vi "Actor Core.vi"(8 "error in":errorcluster, 11 "Example GUI Container in":refnum<class "Example GUI Container.lvclass">) -> (0 "error out":errorcluster, 3 "Actor out":refnum<class "Actor.lvclass">)   [LabVIEW 2023, in "Example GUI View.lvlib" / "Example GUI Container.lvclass"]
doc: "(<B>Filename</B>: Actor Framework.lvlib:Actor.lvclass:Actor Core.vi)\n\nReceives messages to the actor, reacts to them, and initiates any error handling that may shut the actor down.\n\nDescendant classes may override this VI to append parallel tasks for the actor to complete while it handles messages. Overrides use the Call Parent Method node."
uses:
  Example GUI Container.lvclass
  <vilib>/ActorFramework/Actor/Actor.lvclass
  <vilib>/ActorFramework/Actor/Actor.lvclass/Actor.ctl
  <vilib>/ActorFramework/Message Enqueuer/Message Enqueuer.lvclass/Message Enqueuer.ctl
  <vilib>/ActorFramework/Message Enqueuer/Init from Existing Queue.vi
  <vilib>/ActorFramework/Message Enqueuer/Enqueue.vi
  <vilib>/ActorFramework/Stop Msg/Stop Msg.lvclass
  <vilib>/Utility/LVClass/Get LV Class Name.vi
  <resource>/AFDebug/Generate Trace for Message.vi
  <vilib>/ActorFramework/Message Priority Queue/Priority Enqueue.vi
  <vilib>/ActorFramework/Message Enqueuer/Message Enqueuer.lvclass
  GUI Views/GUI Container/GUI Container.lvclass
  GUI Views/GUI Container Messages/Insert View into Subpanel Msg/Insert View into Subpanel Msg.lvclass
  GUI Views/GUI Container Messages/Set View FP State Msg/Set View FP State Msg.lvclass
  GUI Views/GUI Container Messages/Open View FP Msg/Open View FP Msg.lvclass
  GUI Views/GUI Container Messages/Close View FP Msg/Close View FP Msg.lvclass
  GUI Views/GUI Container Messages/Remove View from Subpanel Msg/Remove View from Subpanel Msg.lvclass
panel:
  in  "Remove from Subpanel":bool
  in  "Subpanel":string(combo)
  in  "Close Front Panel":bool
  in  "Activate on Open (F)":bool
  in  "Open Front Panel":bool
  in  "Front Panel State":T1(ring)=enum."Standard"
  in  "Set FP State":bool
  in  "Insert in Subpanel":bool
  in  "Exit":bool
  in  "Views":i32(listbox)
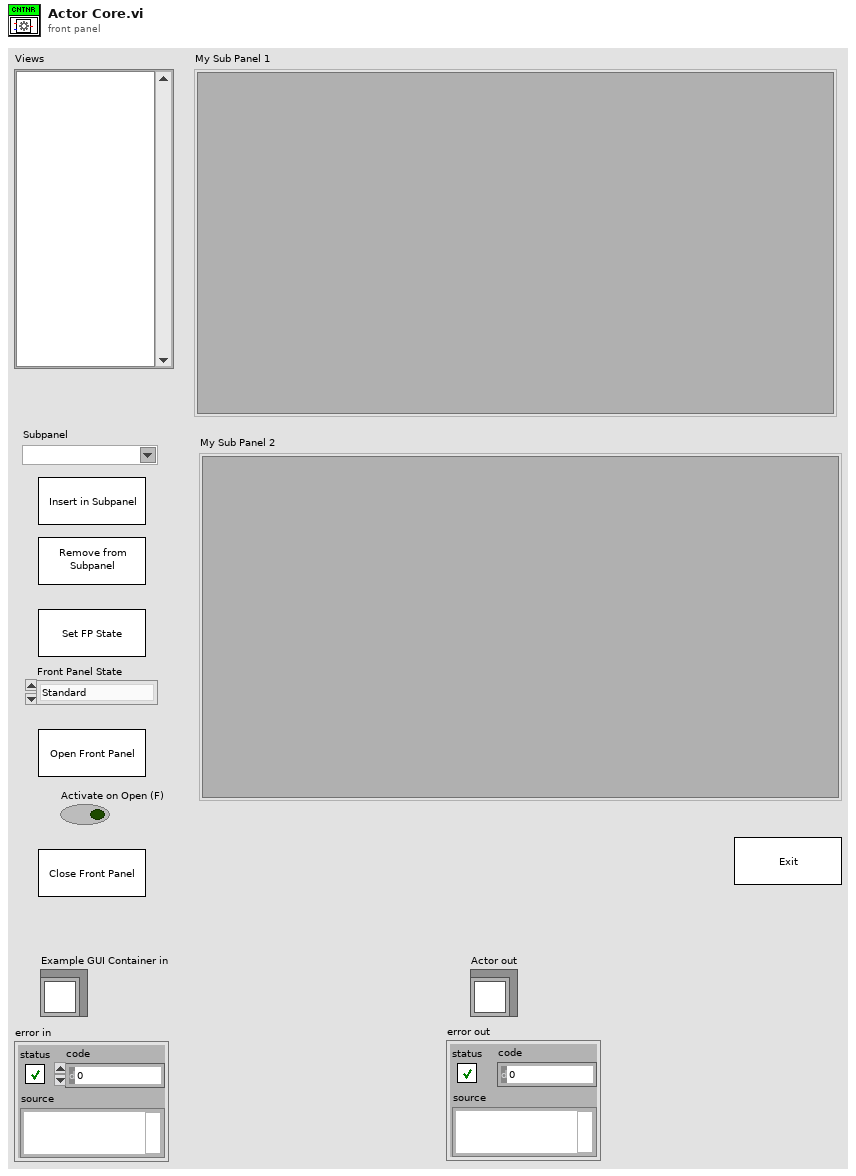
[diagram p1: front panel]
types:
  T1 = enum32{"Invalid", "Standard", "Closed", "Hidden", "Minimized", "Maximized"}
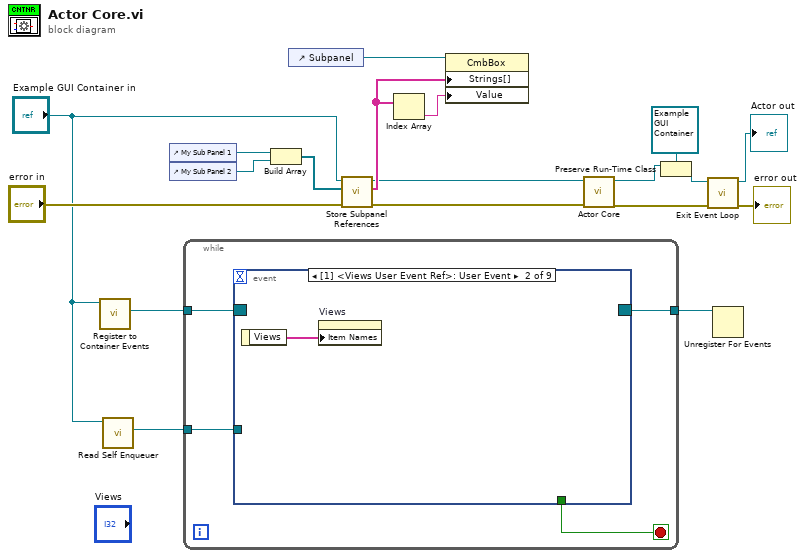
[diagram p0: block diagram]
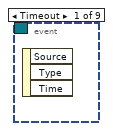
[diagram p2: hidden frame]
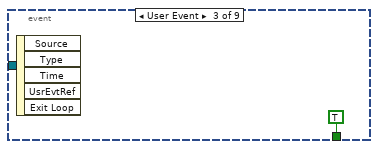
[diagram p3: hidden frame]
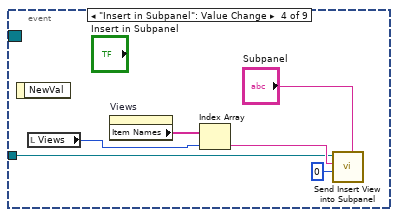
[diagram p4: hidden frame]
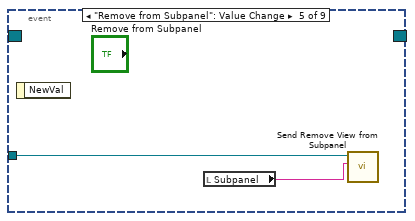
[diagram p5: hidden frame]
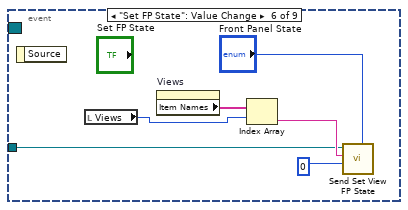
[diagram p6: hidden frame]
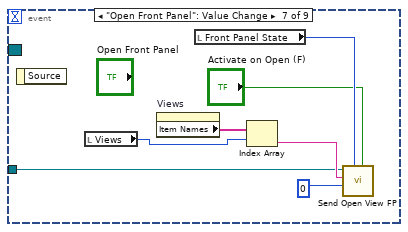
[diagram p7: hidden frame]
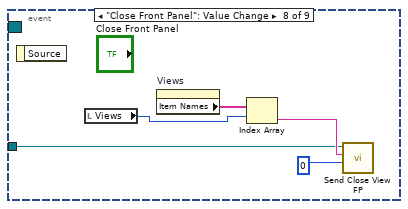
[diagram p8: hidden frame]
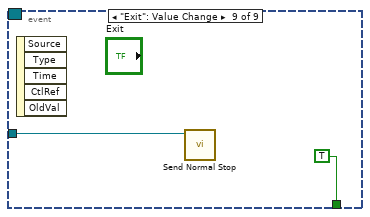
[diagram p9: hidden frame]
diagram:
  n1 = call-dynamic "Register to Container Events.vi"("GUI Container in"="Example GUI Container in") -> ("Event Registration Refnum"=w15:refnum<event-registration>)  [unwired: 8 in, 2 out]
  n2 = call <vilib>:"Read Self Enqueuer.vi"("Actor"="Example GUI Container in") -> ("Self Enqueuer"=w13:refnum<class "Message Enqueuer.lvclass">)  [unwired: 10 in]
  n3 = control-ref of="My Sub Panel 1"() -> (w19:refnum<vi>)
  n4 = control-ref of="My Sub Panel 2"() -> (w11:refnum<vi>)
  n5 = while {
    tunnel: w15 -> [w23]
    tunnel: w13 -> [w22]
    tunnel: [w20] -> w12
    stop <- w21 stop-if-true
    n6 = event shown="[1] <Views User Event Ref>: User Event" {
      selector: w23 -> [_ _ _ _ _ _ _ _ _]
      dyn-events: [_ _ _ _ _ _ _ _ _] -> w20
      timeout: _ -> [_ _ _ _ _ _ _ _ _]
      tunnel: w22 -> [_ _ _ w28 w32 w36 w43 w48 w53]
      tunnel: [_ _ TRUE _ _ _ _ _ TRUE] -> w21
      event Timeout {
        n7 = event-data() -> ()  [unwired: 1 in, 3 out]
      }
      event User Event {
        n8 = event-data() -> ("Views"=w24:string[])  [unwired: 1 in]
        n9 = property on="Views" class="LstBox (strict)"("Item Names"=w24) -> ()  [unwired: 2 in, 2 out]
      }
      event User Event {
        n10 = event-data() -> ()  [unwired: 1 in, 5 out]
      }
      event "Insert in Subpanel": Value Change {
        n11 = event-data() -> ()  [unwired: 1 in, 1 out]
        n12 = local read "Views"() -> (w27:i32)
        n13 = property on="Views" class="LstBox (strict)"() -> ("Item Names"=w31:string[])  [unwired: 2 in, 2 out]
        n14 = Index Array(array=w31, index=w27) -> (element=w30:string)
        n15 = call "Send Insert View into Subpanel.vi"("Subpanel"="Subpanel", "View Hierarchy Level"=0, "View"=w30, "Message Enqueuer in"=w28) -> ()  [unwired: 6 in, 2 out]
      }
      event "Remove from Subpanel": Value Change {
        n16 = event-data() -> ()  [unwired: 1 in, 1 out]
        n17 = local read "Subpanel"() -> (w33:string)
        n18 = call "Send Remove View from Subpanel.vi"("Subpanel"=w33, "Message Enqueuer in"=w32) -> ()  [unwired: 8 in, 2 out]
      }
      event "Set FP State": Value Change {
        n19 = event-data() -> ()  [unwired: 1 in, 1 out]
        n20 = local read "Views"() -> (w34:i32)
        n21 = property on="Views" class="LstBox (strict)"() -> ("Item Names"=w39:string[])  [unwired: 2 in, 2 out]
        n22 = Index Array(array=w39, index=w34) -> (element=w38:string)
        n23 = call "Send Set View FP State.vi"("Front Panel Window:State"="Front Panel State", "View Hierarchy Level"=0, "View"=w38, "Message Enqueuer in"=w36) -> ()  [unwired: 6 in, 2 out]
      }
      event "Open Front Panel": Value Change {
        n24 = event-data() -> ()  [unwired: 1 in, 1 out]
        n25 = local read "Views"() -> (w42:i32)
        n26 = property on="Views" class="LstBox (strict)"() -> ("Item Names"=w46:string[])  [unwired: 2 in, 2 out]
        n27 = local read "Front Panel State"() -> (w41:T1)
        n28 = Index Array(array=w46, index=w42) -> (element=w45:string)
        n29 = call "Send Open View FP.vi"("Activate on Open (F)"="Activate on Open (F)", "State On Open (Standard)"=w41, "View Hierarchy Level"=0, "View"=w45, "Message Enqueuer in"=w43) -> ()  [unwired: 5 in, 2 out]
      }
      event "Close Front Panel": Value Change {
        n30 = event-data() -> ()  [unwired: 1 in, 1 out]
        n31 = local read "Views"() -> (w47:i32)
        n32 = property on="Views" class="LstBox (strict)"() -> ("Item Names"=w51:string[])  [unwired: 2 in, 2 out]
        n33 = Index Array(array=w51, index=w47) -> (element=w50:string)
        n34 = call "Send Close View FP.vi"("View Hierarchy Level"=0, "View"=w50, "Message Enqueuer in"=w48) -> ()  [unwired: 7 in, 2 out]
      }
      event "Exit": Value Change {
        n35 = event-data() -> ()  [unwired: 1 in, 5 out]
        n36 = call <vilib>:"Send Normal Stop.vi"("Message Enqueuer"=w53) -> ()  [unwired: 10 in, 1 out]
      }
    }
  }
  n37 = Build Array(w19, w11) -> (w18:refnum<vi>[])
  n38 = control-ref of="Subpanel"() -> (w10:refnum<vi>)
  n39 = call "Store Subpanel References.vi"("error in (no error)"="error in", "Subpanel References"=w18, "GUI Container in"="Example GUI Container in") -> ("error out"=w16:errorcluster, "Sub Panel Names"=w9:string[], "GUI Container out"=w6:refnum<class "Example GUI Container.lvclass">)  [unwired: 6 in]
  n40 = Index Array(array=w9) -> (element=w8:string)  [unwired: 1 in]
  n41 = property class="CmbBox"(reference=w10, "Strings[]"=w9, "Value"=w8) -> ()  [unwired: 1 in, 2 out]
  n42 = call-parent "Actor Core.vi"("error in"=w16, "GUI View in"=w6) -> ("error out"=w4:errorcluster, "Actor out"=w7:refnum<class "Actor.lvclass">)  [unwired: 8 in]
  n43 = Preserve Run-Time Class(object in=w7, 2:refnum<class "Example GUI Container.lvclass"> refnum ("Example GUI Container in")) -> (object out=w5:refnum<class "Example GUI Container.lvclass">)  [unwired: 1 in, 1 out]
  n44 = call "Exit Event Loop.vi"("error in (no error)"=w4, "GUI Container in"=w5) -> ("error out"=→"error out":errorcluster, "GUI Container out"=→"Actor out":refnum<class "Example GUI Container.lvclass">)  [unwired: 8 in]
  n45 = Unregister For Events(event registration refnum=w12) -> ()  [unwired: 1 in, 1 out]
